vi "Read Controller Activity.vi"(4 "error in (no error)":errorcluster, 7 "VISA resource name":refnum<visa-resource-name>) -> (0 "error out":errorcluster, 2 "Controller Activity":T1, 3 "VISA resource name out":refnum<visa-resource-name>)   [LabVIEW 2019, in "Newport ESP301.lvlib"]
doc: "Reads the controller activity."
uses:
  Newport ESP301.lvlib
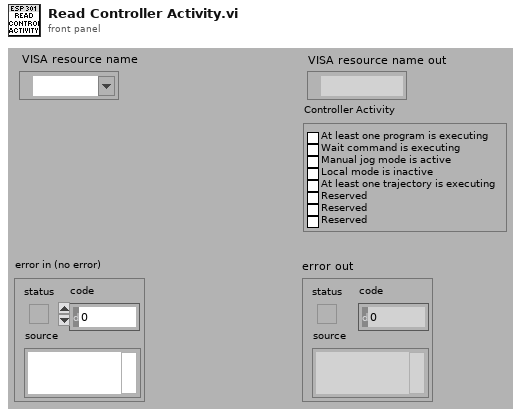
[diagram p1: front panel]
types:
  T1 = cluster{"At least one program is executing":bool, "Wait command is executing":bool, "Manual jog mode is active":bool, "Local mode is inactive":bool, "At least one trajectory is executing":bool, "Reserved":bool, "Reserved":bool, "Reserved":bool}
  T2 = cluster{"Boolean array[0]":bool, "Boolean array[1]":bool, "Boolean array[2]":bool, "Boolean array[3]":bool, "Boolean array[4]":bool, "Boolean array[5]":bool, "Boolean array[6]":bool, "Boolean array[7]":bool}
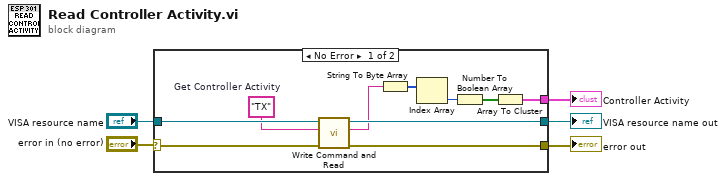
[diagram p0: block diagram]
diagram:
  n1 = case shown="No Error" "error in (no error)" {
    selector: "error in (no error)" -> [w14 w17]
    tunnel: [w13 w17] -> w4
    tunnel: "VISA resource name" -> [w15 w16]
    tunnel: [w12 w16] -> w2
    tunnel: [w7 _] -> w1
    frame No Error {
      w6 = "TX"  # Get Controller Activity
      n2 = call "Write Command and Read.vi"("error in (no error)"=w14, "Command"=w6, "VISA resource name"=w15) -> ("error out"=w13:errorcluster, "Returned string"=w11:string, "VISA resource name out"=w12:refnum<visa-resource-name>)  [unwired: 4 in]
      n3 = String To Byte Array(string=w11) -> (unsigned byte array=w10:u8[])
      n4 = Index Array(array=w10) -> (element=w9:u8)  [unwired: 1 in]
      n5 = Number To Boolean Array(number=w9) -> (Boolean array=w8:bool[])
      n6 = Array To Cluster(array=w8) -> (cluster=w7:T2)
    }
    frame Error {
    }
  }
  "error out" <- w4
  "VISA resource name out" <- w2
  "Controller Activity" <- w1
